vi "SetPort.vi"(8 "error in":errorcluster, 10 "Slit":string, 11 "Port":refnum<visa-resource-name>) -> (0 "error out":errorcluster, 2 "String":string, 3 "Port out":refnum<visa-resource-name>)   [LabVIEW 2018]
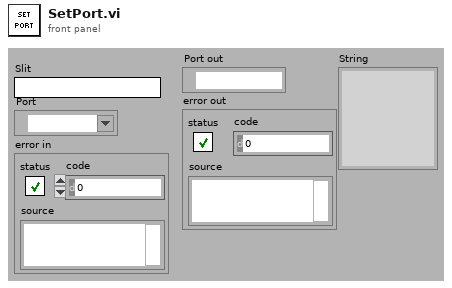
[diagram p1: front panel]
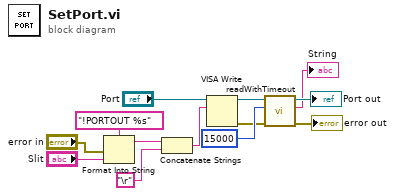
[diagram p0: block diagram]
diagram:
  n1 = Format Into String(format string="!PORTOUT %s" ("concatenated string"), error in="error in", "Slit") -> (resulting string=w11:string)  [unwired: 1 in, 1 out]
  n2 = Concatenate Strings(w11, "\r") -> (w8:string)
  n3 = VISA Write(VISA resource name="Port", write buffer=w8) -> (VISA resource name out=w5:refnum<visa-resource-name>, error out=w3:errorcluster)  [unwired: 1 in, 1 out]
  n4 = call "readWithTimeout.vi"("error in"=w3, "timeOut"=u32 15000, "Port"=w5) -> ("error out"=→"error out":errorcluster, "String"=→"String":string, "Port out"=→"Port out":refnum<visa-resource-name>)  [unwired: 6 in]
